vi "DAQmx.44xx.Configure Trigger.vi"(8 "error in (no error)":errorcluster, 10 "master task in":refnum<k21>, 11 "task in":refnum<k21>) -> (0 "error out":errorcluster, 3 "task out":refnum<k21>)   [LabVIEW 2019, in "DAQmx.lvclass"]
uses:
  DAQmx.lvclass
  <vilib>/DAQmx/configure/trigger.llb/DAQmx Start Trigger (Digital Edge).vi
  <resource>/objmgr/daqmx.rc
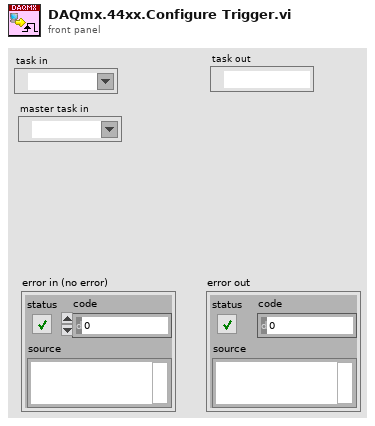
[diagram p1: front panel]
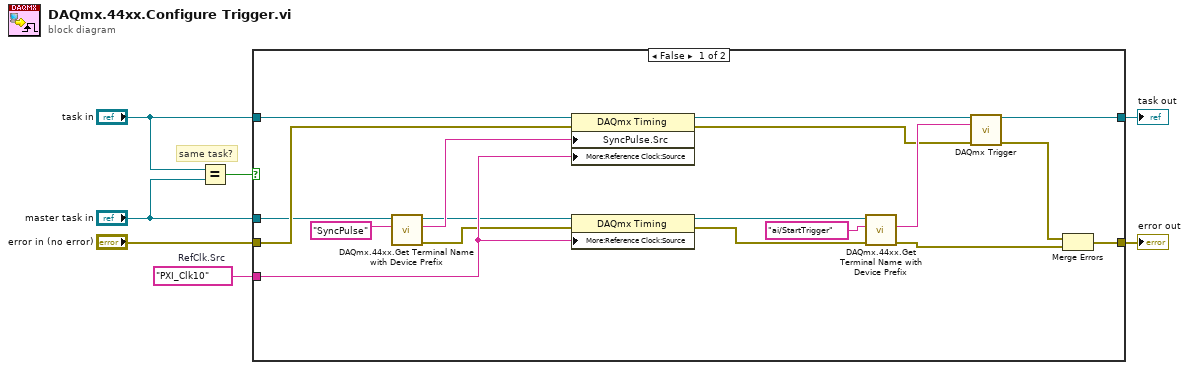
[diagram p0: block diagram]
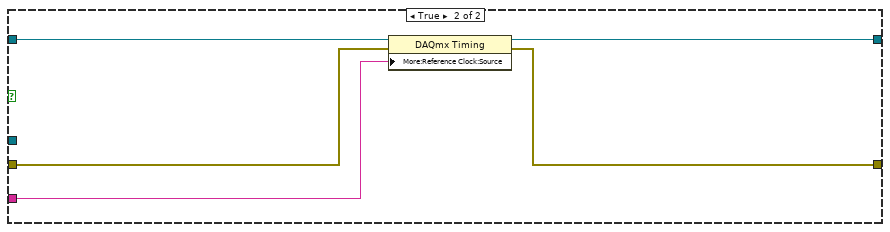
[diagram p2: hidden frame]
diagram:
  w1 = tag "PXI_Clk10"  # RefClk.Src
  # "same task?"
  n1 = Equal?(x="task in", y="master task in") -> (x = y?=w2:bool)
  n2 = case shown="False" w2 {
    tunnel: "error in (no error)" -> [w12 w29]
    tunnel: [w21 w28] -> w6
    tunnel: [w15 w27] -> w5
    tunnel: "master task in" -> [w8 _]
    tunnel: "task in" -> [w23 w30]
    tunnel: w1 -> [w11 w26]
    frame False {
      n3 = call "DAQmx.44xx.Get Terminal Name with Device Prefix.vi"("Local Terminal Name"="SyncPulse", "task"=w8) -> ("error out"=w9:errorcluster, "Terminal Name with Device Prefix"=w17:tag, "task out"=w10:refnum<k21>)  [unwired: 7 in]
      n4 = property class="DAQmx Timing"(reference=w23, error in=w12, "SyncPulse.Src"=w17, "More:Reference Clock:Source"=w11) -> (reference out=w22:refnum<k21>, error out=w19:errorcluster)
      n5 = property class="DAQmx Timing"(reference=w10, error in=w9, "More:Reference Clock:Source"=w11) -> (reference out=w13:refnum<k21>, error out=w18:errorcluster)
      n6 = call "DAQmx.44xx.Get Terminal Name with Device Prefix.vi"("error in (no error)"=w18, "Local Terminal Name"="ai/StartTrigger", "task"=w13) -> ("error out"=w14:errorcluster, "Terminal Name with Device Prefix"=w20:tag)  [unwired: 6 in, 1 out]
      n7 = call-poly <vilib>:"DAQmx Trigger.vi"("task/channels in"=w22, "source"=w20, "error in"=w19) -> ("task out"=w21:refnum<k21>, "error out"=w16:errorcluster)  [unwired: 11 in]
      n8 = Merge Errors(w16, w14) -> (w15:errorcluster)
    }
    frame True {
      n9 = property class="DAQmx Timing"(reference=w30, error in=w29, "More:Reference Clock:Source"=w26) -> (reference out=w28:refnum<k21>, error out=w27:errorcluster)
    }
  }
  "error out" <- w5
  "task out" <- w6
